vi "ZREM.vi"(0 "TCP session out":refnum<k5>, 1 "Key":string, 5 "Members":string[](array[string]), 11 "error in":errorcluster) -> (4 "TCP session out":refnum<k5>, 6 "Data":T1, 15 "error out":errorcluster)   [LabVIEW 2023]
uses:
  SubVIs/Controls/redis-data.ctl
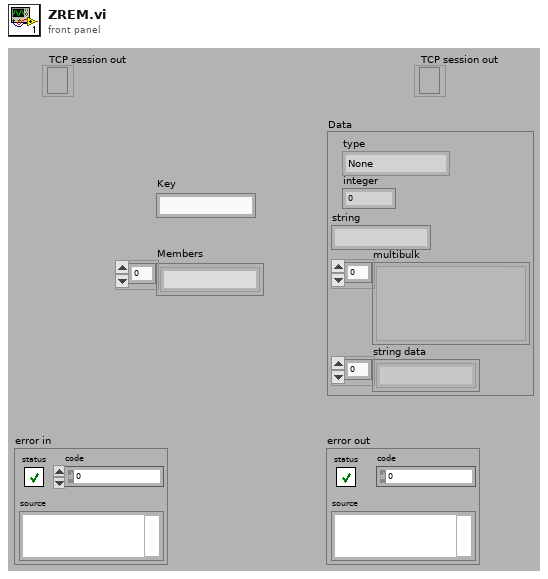
[diagram p1: front panel]
types:
  T1 = typedef "redis-data.ctl" = cluster{"type":enum16{"None", "Error", "Status", "Nil", "Integer", "String", "Multibulk"}, "integer":i64, "string":string, "multibulk":variant[], "string data":string[]}
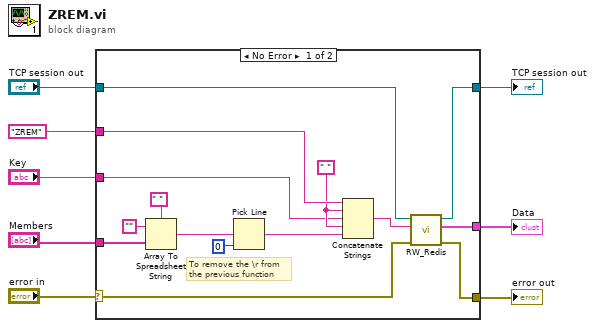
[diagram p0: block diagram]
diagram:
  n1 = case shown="No Error" "error in" {
    selector: "error in" -> [w16 w25]
    tunnel: "Members" -> [w23 _]
    tunnel: "ZREM" -> [w13 _]
    tunnel: "TCP session out" -> [w10 w24]
    tunnel: [w15 w25] -> w5
    tunnel: [w14 _] -> w1
    tunnel: "Key" -> [w11 _]
    tunnel: [w9 w24] -> w2
    frame No Error {
      w12 = " "
      # "To remove the \\r from\nthe previous function"
      n2 = Array To Spreadsheet String(delimiter (Tab)=" ", array=w23, 3:"" ("format string")) -> (spreadsheet string=w19:string)
      n3 = Pick Line(multi-line string=w19, line index=0) -> (output string=w20:string)  [unwired: 1 in]
      n4 = Concatenate Strings(w13, w12, w11, w12, w20) -> (w17:string)
      n5 = call "RW_Redis.vi"("error in"=w16, "command"=w17, "TCP session in"=w10) -> ("error out"=w15:errorcluster, "Data"=w14:T1, "TCP session out"=w9:refnum<k5>)  [unwired: 6 in]
    }
    frame Error {
    }
  }
  "error out" <- w5
  "TCP session out" <- w2
  "Data" <- w1
